vi "pdbm_TaskRoute_service.vi"(8 "error in (no error)":errorcluster, 10 "TaskDisplay":refnum<vi>, 11 "pdbm_testsys_event":T1) -> ()   [LabVIEW 2015]
doc: "handles message between pdbm_testsystem and tasks.\n-------------------------------------------------------------------\nAuthor: Dang Lam\nCreated: Feb, 10, 2012"
uses:
  pdbm_testsys_taskroute_inter/UsrDefine/pdbm_testsys_reqst_data.ctl
  test_system/UsrDefine/pdbm_testsystem_feedback_data.ctl
  test_system/public/getTaskInfo_byRef.vi
  pdbm_test_route/pdbm_task_route.lvlib
  test_system/pdbm_test_system.lvlib
  pdbm_testsys_taskroute_inter/pdbm_testsys_taskroute_inter.lvlib
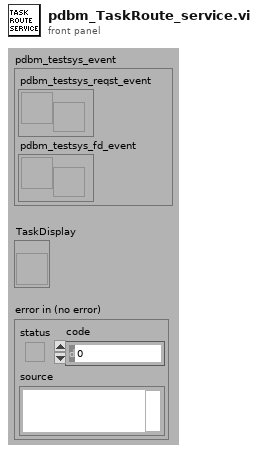
[diagram p1: front panel]
types:
  T1 = cluster{"pdbm_testsys_reqst_event":refnum<user-event>, "pdbm_testsys_fd_event":refnum<user-event>}
  T2 = cluster{"pdbm_testsys_reg_reqst_event":refnum<event-registration>, "pdbm_taskroute_reg_fd_event":refnum<event-registration>}
  T3 = cluster{"pdbm_testsys_fd_event":refnum<user-event>, "pdbm_testsys_reqst_event":refnum<user-event>, "pdbm_taskroute_fd_event":refnum<user-event>}
  T4 = cluster{"TaskName":string, "TaskRef":refnum<vi>}[]
  T5 = enum32{"Invalid", "Standard", "Closed", "Hidden", "Minimized", "Maximized"}
  T6 = typedef "pdbm_test_route.lvlib/TaskFeedbackCmd.ctl" = cluster{"TaskRef":refnum<vi>, "Command":string, "Variant":variant}
  T7 = typedef "pdbm_testsys_taskroute_inter.lvlib/pdbm_testsys_reqst_data.ctl" = cluster{"TaskName":string, "Request":string, "Data":variant}
  T8 = cluster{"pdbm_taskroute_fd_event":refnum<user-event>, "Data":variant}
  T9 = cluster{"TaskName":string, "Task Ref":refnum<vi>}
  T10 = cluster{"TaskName":string, "Task Ref":refnum<vi>}[]
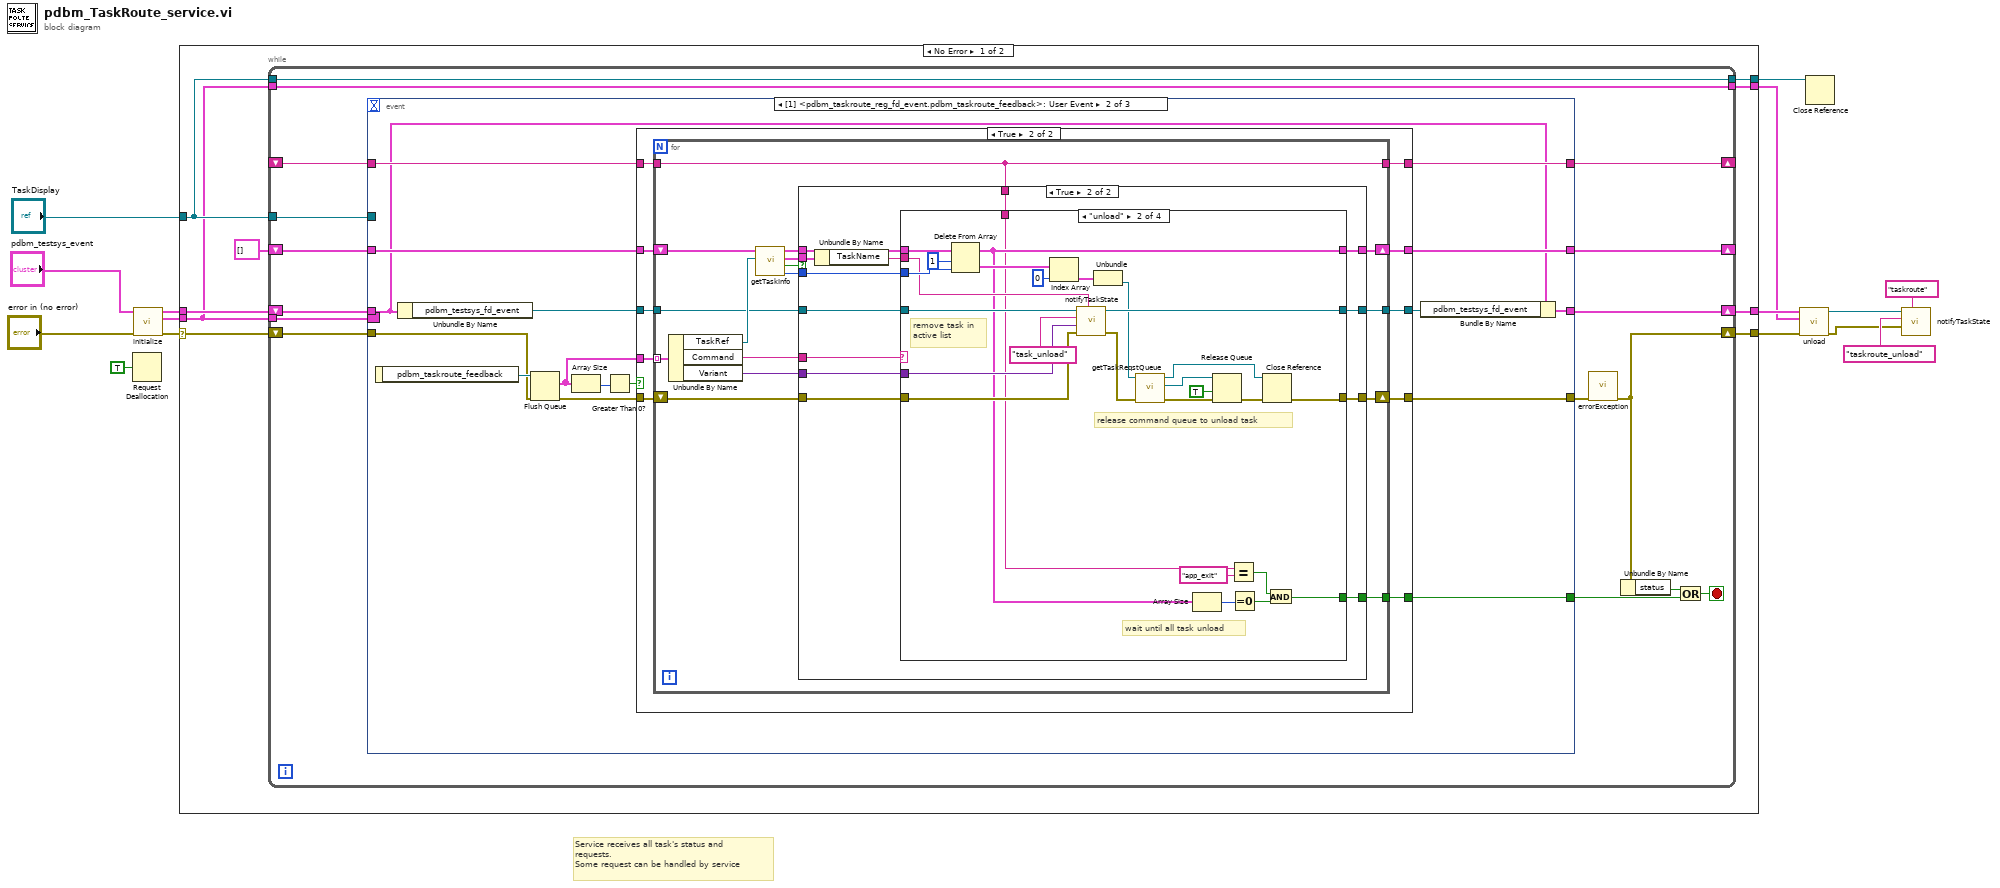
[diagram p0: block diagram]
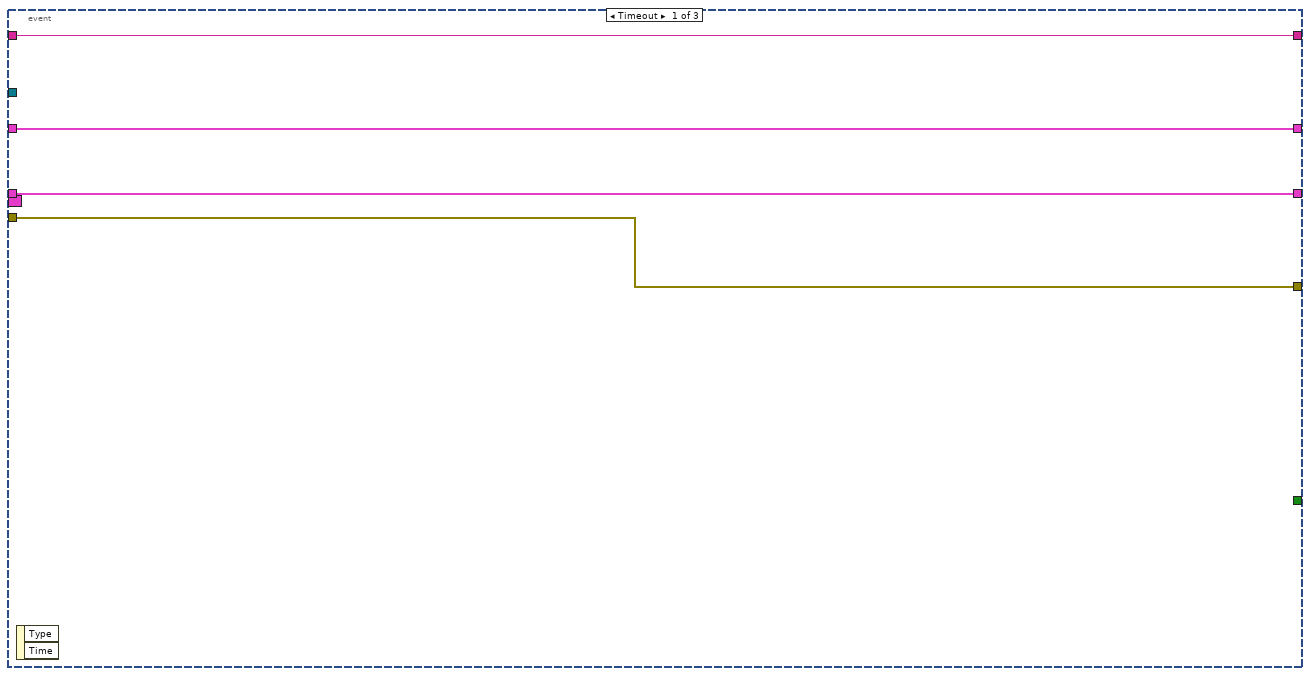
[diagram p2: hidden frame]
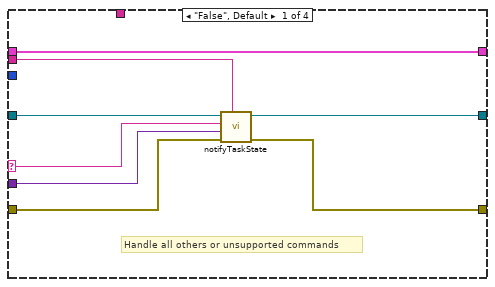
[diagram p5: hidden frame]
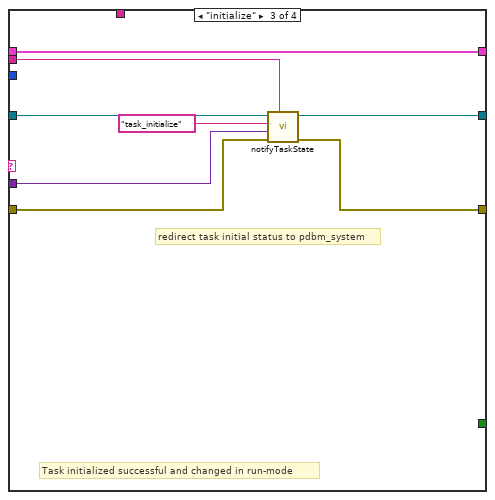
[diagram p6: hidden frame]
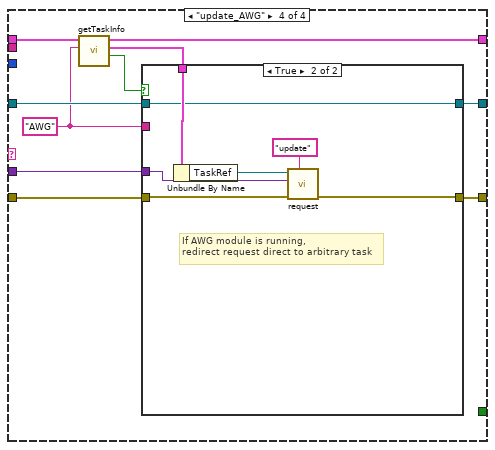
[diagram p7: hidden frame]
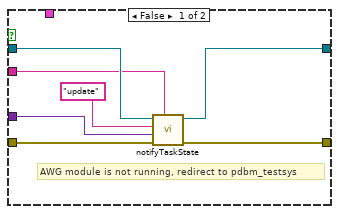
[diagram p8: hidden frame]
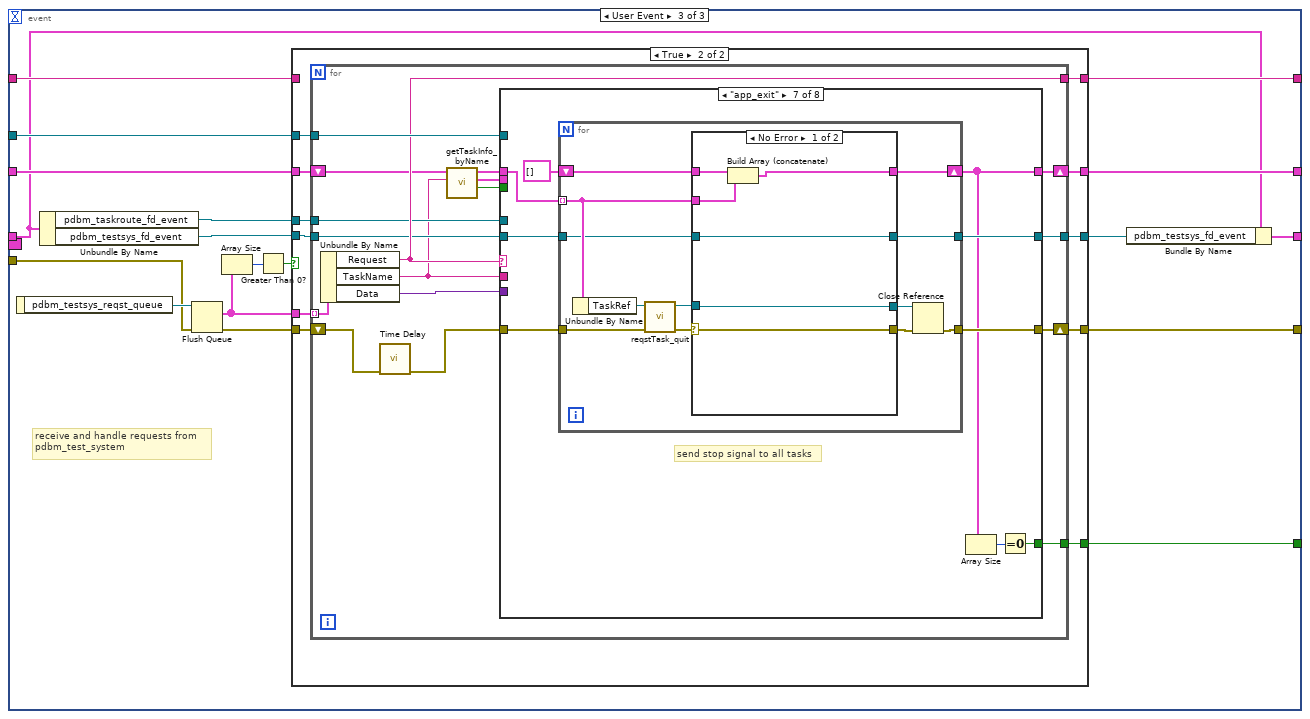
[diagram p9: hidden frame]
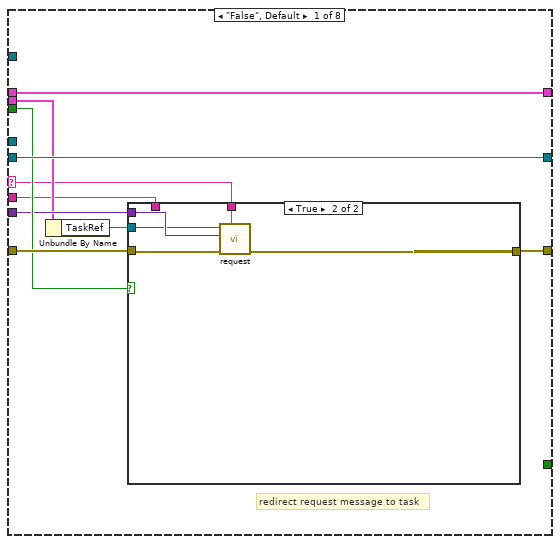
[diagram p11: hidden frame]
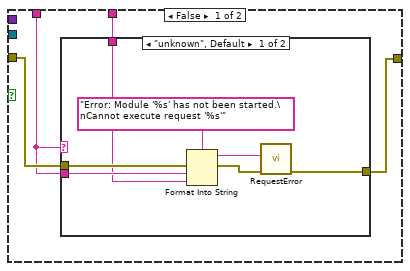
[diagram p12: hidden frame]
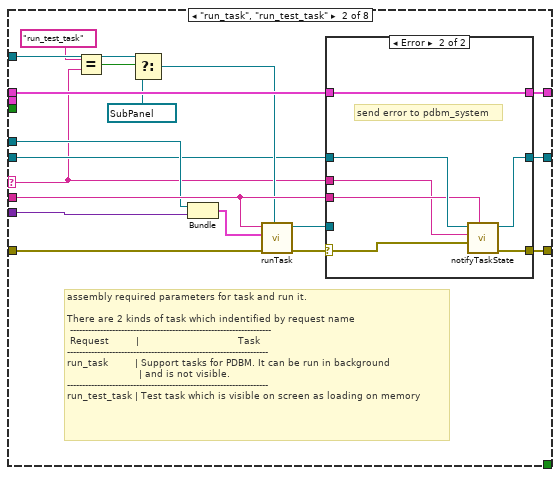
[diagram p14: hidden frame]
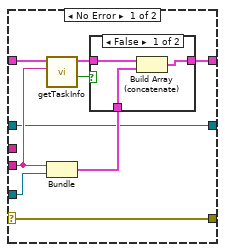
[diagram p15: hidden frame]
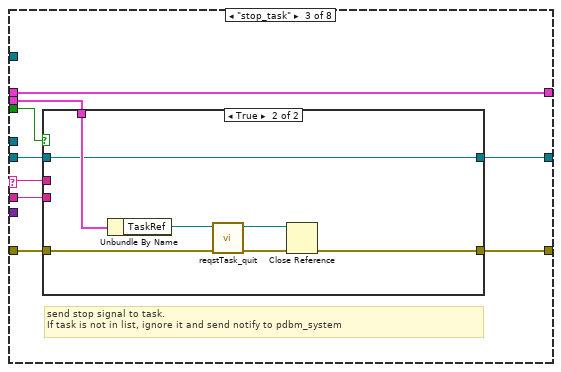
[diagram p17: hidden frame]
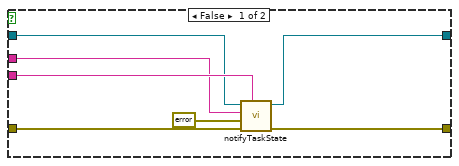
[diagram p18: hidden frame]
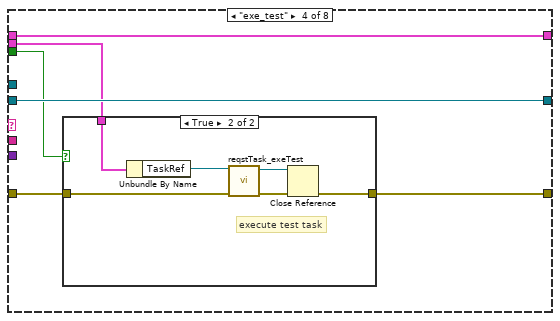
[diagram p19: hidden frame]
diagram:
  # "Service receives all task's status and\nrequests.\nSome request can be handled by service"
  n1 = Request Deallocation(TRUE ("flag")) -> ()
  n2 = call "initialize.vi"("error in (no error)"="error in (no error)", "pdbm_testsys_event"="pdbm_testsys_event") -> ("error IO"=w15:errorcluster, "pdbm_taskroute_reg_event"=w13:T2, "pdbm_taskroute_event"=w14:T3)  [unwired: 7 in]
  n3 = case shown="No Error" w15 {
    selector: w15 -> [w24 w381]
    tunnel: w14 -> [w21 w380]
    tunnel: w13 -> [w16 w379]
    tunnel: "TaskDisplay" -> [w20 w382]
    tunnel: [w19 w382] -> w2
    tunnel: [w22 w381] -> w7
    tunnel: [w18 w380] -> w6
    tunnel: [w17 w379] -> w5
    frame No Error {
      n4 = while {
        shift-right: [w27] -> w22
        shift-left: w24 -> [w40]
        tunnel: w16 -> [w39]
        shift-right: [w37] -> _
        shift-left: T4 [] -> [w38]
        tunnel: w20 -> [w36]
        shift-right: [w35] -> _
        shift-left: _ -> [w34]
        tunnel: w20 -> [w33]
        tunnel: [w33] -> w19
        shift-right: [w28] -> w18
        shift-left: w21 -> [w26]
        tunnel: [w25] -> w17
        tunnel: w16 -> [w25]
        stop <- w30 stop-if-true
        n5 = event shown="[1] <pdbm_taskroute_reg_fd_event.pdbm_taskroute_feedback>: User Event" {
          selector: w39 -> [_ _ _]
          dyn-events: _ -> [_ _ _]
          timeout: _ -> [_ _ _]
          tunnel: w40 -> [w43 w59 w190]
          tunnel: [w43 w58 w188] -> w32
          tunnel: w38 -> [w44 w57 w187]
          tunnel: [w44 w56 w186] -> w37
          tunnel: w36 -> [_ _ w185]
          tunnel: [w42 w54 w184] -> w35
          tunnel: w34 -> [w42 w55 w180]
          tunnel: [_ w53 w179] -> w31
          tunnel: w26 -> [w41 w47 w177]
          tunnel: [w41 w46 w175] -> w28
          event Timeout {
            n6 = event-data() -> ()  [unwired: 1 in, 2 out]
          }
          event User Event {
            n7 = event-data() -> ("pdbm_taskroute_feedback"=w60:refnum<queue>)  [unwired: 1 in]
            n8 = Unbundle By Name(w47) -> ("pdbm_testsys_fd_event"=w52:refnum<user-event>)
            n9 = Flush Queue(queue=w60, error in (no error)=w59) -> (remaining elements=w51:T6[], error out=w48:errorcluster)  [unwired: 1 out]
            n10 = Array Size(array=w51) -> (size(s)=w49:i32)
            n11 = Greater Than 0?(x=w49) -> (x > 0?=w50:bool)
            n12 = case shown="True" w50 {
              tunnel: w51 -> [_ w74]
              tunnel: [w61 w73] -> w58
              tunnel: w57 -> [w63 w72]
              tunnel: [w63 w71] -> w56
              tunnel: w55 -> [w64 w70]
              tunnel: [w64 w69] -> w54
              tunnel: [_ w68] -> w53
              tunnel: w52 -> [w62 w67]
              tunnel: [w62 w66] -> w45
              tunnel: w48 -> [w61 w65]
              frame False {
              }
              frame True {
                n13 = for {
                  tunnel: w74 -> [w89] mode=indexing
                  shift-right: [w80] -> w73
                  shift-left: w65 -> [w75]
                  shift-right: [w81] -> w71
                  shift-left: w72 -> [w90]
                  tunnel: w70 -> [w79]
                  tunnel: [w79] -> w69
                  tunnel: [w78] -> w68
                  tunnel: w67 -> [w77]
                  tunnel: [w76] -> w66
                  n14 = Unbundle By Name(w89) -> ("TaskRef"=w88:refnum<vi>, "Command"=w83:string, "Variant"=w82:variant)
                  n15 = call-poly "getTaskInfo.vi"("TaskRef in"=w88, "ActiveTask in"=w90) -> ("index"=w84:i32, "found?"=w87:bool, "TaskInfo"=w85:cluster{"TaskName":string, "TaskRef":refnum<vi>}, "ActiveTask out"=w86:T4)  [unwired: 6 in]
                  n16 = case shown="True" w87 {
                    tunnel: w86 -> [w93 w106]
                    tunnel: w85 -> [_ w95]
                    tunnel: w84 -> [_ w104]
                    tunnel: w83 -> [_ w105]
                    tunnel: w82 -> [_ w102]
                    tunnel: [w93 w103] -> w81
                    tunnel: w75 -> [w92 w101]
                    tunnel: [w92 w100] -> w80
                    tunnel: w79 -> [_ w99]
                    tunnel: [_ w98] -> w78
                    tunnel: w77 -> [w91 w97]
                    tunnel: [w91 w96] -> w76
                    frame False {
                    }
                    frame True {
                      n17 = Unbundle By Name(w95) -> ("TaskName"=w94:string)
                      n18 = case shown="\"unload\"" w105 {
                        selector: w105 -> [w110 _ _ _]
                        tunnel: w106 -> [w114 w141 w149 w159]
                        tunnel: w104 -> [_ w140 _ _]
                        tunnel: [w114 w116 w149 w158] -> w103
                        tunnel: w102 -> [w112 w133 w148 w152]
                        tunnel: [w109 w119 w146 w153] -> w100
                        tunnel: w101 -> [w111 w134 w147 w154]
                        tunnel: w99 -> [_ w115 _ _]
                        tunnel: [_ w136 _ _] -> w98
                        tunnel: w97 -> [w113 w135 w145 w156]
                        tunnel: w94 -> [w107 w130 w142 _]
                        tunnel: [w108 w131 w143 w151] -> w96
                        frame "False", Default {
                          # "Handle all others or unsupported commands"
                          n19 = call "notifyTaskState.vi"("TaskName"=w107, "error in (no error)"=w111, "Data"=w112, "Request"=w110, "pdbm_testsystem_feeback_event"=w113) -> ("error out"=w109:errorcluster, "pdbm_testsystem_feeback_event out"=w108:refnum<user-event>)  [unwired: 5 in]
                        }
                        frame "unload" {
                          # "release command queue to unload task"
                          # "remove task in\nactive list"
                          # "wait until all task unload"
                          n20 = Delete From Array(array=w141, length=1, index=w140) -> (deleted portion=w124:T4, array with subset deleted=w116:T4)
                          n21 = Index Array(array=w124, index=0) -> (element=w125:cluster{"TaskName":string, "TaskRef":refnum<vi>})
                          n22 = call "notifyTaskState.vi"("TaskName"=w130, "error in (no error)"=w134, "Data"=w133, "Request"="task_unload", "pdbm_testsystem_feeback_event"=w135) -> ("error out"=w126:errorcluster, "pdbm_testsystem_feeback_event out"=w131:refnum<user-event>)  [unwired: 5 in]
                          n23 = Unbundle(w125) -> ("TaskRef"=w123:refnum<vi>)  [unwired: 1 out]
                          n24 = call "getTaskReqstQueue.vi"("error in (no error)"=w126, "TaskRef"=w123) -> ("error IO"=w122:errorcluster, "TaskReqst_queue"=w121:refnum<queue>, "TaskRef out"=w118:refnum<vi>)  [unwired: 7 in]
                          n25 = Array Size(array=w116) -> (size(s)=w137:i32)
                          n26 = Release Queue(queue=w121, force destroy? (F)=TRUE, error in (no error)=w122) -> (error out=w120:errorcluster)  [unwired: 2 out]
                          n27 = Equal?(x=w115, y="app_exit") -> (x = y?=w127:bool)
                          n28 = Equal To 0?(x=w137) -> (x = 0?=w128:bool)
                          n29 = Close Reference(reference=w118, error in (no error)=w120) -> (error out=w119:errorcluster)
                          n30 = And(x=w127, y=w128) -> (x .and. y?=w136:bool)
                        }
                        frame "initialize" {
                          # "redirect task initial status to pdbm_system"
                          # "Task initialized successful and changed in run-mode"
                          n31 = call "notifyTaskState.vi"("TaskName"=w142, "error in (no error)"=w147, "Data"=w148, "Request"="task_initialize", "pdbm_testsystem_feeback_event"=w145) -> ("error out"=w146:errorcluster, "pdbm_testsystem_feeback_event out"=w143:refnum<user-event>)  [unwired: 5 in]
                        }
                        frame "update_AWG" {
                          w150 = "AWG" ("TaskName")
                          n32 = call-poly "getTaskInfo.vi"("TaskName"=w150, "ActiveTask in"=w159) -> ("found?"=w157:bool, "TaskInfo"=w155:cluster{"TaskName":string, "TaskRef":refnum<vi>}, "ActiveTask out"=w158:T4)  [unwired: 6 in, 1 out]
                          n33 = case shown="True" w157 {
                            tunnel: w156 -> [w166 w167]
                            tunnel: w155 -> [_ w170]
                            tunnel: w154 -> [w164 w173]
                            tunnel: [w163 w172] -> w153
                            tunnel: w152 -> [w160 w168]
                            tunnel: [w165 w167] -> w151
                            tunnel: w150 -> [w162 _]
                            frame False {
                              # "AWG module is not running, redirect to pdbm_testsys"
                              n34 = call "notifyTaskState.vi"("TaskName"=w162, "error in (no error)"=w164, "Data"=w160, "Request"="update", "pdbm_testsystem_feeback_event"=w166) -> ("error out"=w163:errorcluster, "pdbm_testsystem_feeback_event out"=w165:refnum<user-event>)  [unwired: 5 in]
                            }
                            frame True {
                              # "If AWG module is running,\nredirect request direct to arbitrary task"
                              n35 = Unbundle By Name(w170) -> ("TaskRef"=w169:refnum<vi>)
                              n36 = call "request.vi"("request"="update", "error in (no error)"=w173, "Parameter"=w168, "TaskRef in"=w169) -> ("error IO"=w172:errorcluster)  [unwired: 6 in, 1 out]
                            }
                          }
                        }
                      }
                    }
                  }
                }
              }
            }
            n37 = Bundle By Name(cluster=w47, "pdbm_testsys_fd_event"=w45) -> (w46:T3)
          }
          event User Event {
            # "receive and handle requests from\npdbm_test_system"
            n38 = event-data() -> ("pdbm_testsys_reqst_queue"=w191:refnum<queue>)  [unwired: 1 in]
            n39 = Unbundle By Name(w177) -> ("pdbm_taskroute_fd_event"=w174:refnum<user-event>, "pdbm_testsys_fd_event"=w178:refnum<user-event>)
            n40 = Flush Queue(queue=w191, error in (no error)=w190) -> (remaining elements=w183:T7[], error out=w189:errorcluster)  [unwired: 1 out]
            n41 = Array Size(array=w183) -> (size(s)=w182:i32)
            n42 = Greater Than 0?(x=w182) -> (x > 0?=w181:bool)
            n43 = case shown="True" w181 {
              tunnel: w189 -> [w193 w206]
              tunnel: [w193 w205] -> w188
              tunnel: w178 -> [w192 w204]
              tunnel: w187 -> [w194 w203]
              tunnel: [w194 w202] -> w186
              tunnel: w185 -> [_ w201]
              tunnel: [w195 w200] -> w184
              tunnel: w183 -> [_ w199]
              tunnel: w180 -> [w195 _]
              tunnel: [_ w198] -> w179
              tunnel: [w192 w197] -> w176
              tunnel: w174 -> [_ w196]
              frame False {
              }
              frame True {
                n44 = for {
                  tunnel: w199 -> [w223] mode=indexing
                  shift-right: [w221] -> w205
                  shift-left: w206 -> [w208]
                  tunnel: w204 -> [w216]
                  shift-right: [w220] -> w202
                  shift-left: w203 -> [w213]
                  tunnel: w201 -> [w219]
                  tunnel: [w218] -> w200
                  tunnel: [w217] -> w198
                  tunnel: [w215] -> w197
                  tunnel: w196 -> [w214]
                  n45 = Unbundle By Name(w223) -> ("Request"=w218:string, "TaskName"=w211:string, "Data"=w222:variant)
                  n46 = call "Time Delay"("error in (no error)"=w208) -> ("error out"=w207:errorcluster)  [unwired: 10 in]
                  n47 = call "getTaskInfo_byName.vi"("TaskName"=w211, "ActiveTask in"=w213) -> ("found?"=w209:bool, "TaskInfo"=w210:cluster{"TaskName":string, "TaskRef":refnum<vi>}, "ActiveTask out"=w212:T4)  [unwired: 6 in, 1 out]
                  n48 = case shown="\"app_exit\"" w218 {
                    selector: w218 -> [w225 w251 w294 _ _ _ _ _]
                    tunnel: w216 -> [w233 w253 w293 w315 w325 w328 w334 w367]
                    tunnel: w207 -> [w231 w268 w297 w317 w327 w330 w339 w371]
                    tunnel: w211 -> [w224 w263 w295 _ _ _ _ _]
                    tunnel: w222 -> [w229 w267 _ _ _ _ _ _]
                    tunnel: [w228 w265 w296 w316 w327 w330 w338 w370] -> w221
                    tunnel: w212 -> [w232 w264 w291 w314 w326 w329 w335 w369]
                    tunnel: [w232 w261 w291 w314 w326 w329 w332 w368] -> w220
                    tunnel: w219 -> [_ w260 _ _ _ _ _ _]
                    tunnel: [_ _ _ _ _ _ w336 _] -> w217
                    tunnel: [w233 w252 w292 w315 w325 w328 w333 w367] -> w215
                    tunnel: w214 -> [_ w254 _ _ _ _ _ _]
                    tunnel: w210 -> [w227 _ w290 w313 _ _ _ _]
                    tunnel: w209 -> [w230 _ w289 w312 _ _ _ _]
                    frame "False", Default {
                      # "redirect request message to task"
                      n49 = Unbundle By Name(w227) -> ("TaskRef"=w226:refnum<vi>)
                      n50 = case shown="True" w230 {
                        tunnel: w231 -> [w237 w250]
                        tunnel: w229 -> [_ w248]
                        tunnel: [w235 w249] -> w228
                        tunnel: w226 -> [_ w247]
                        tunnel: w225 -> [w236 w246]
                        tunnel: w224 -> [w234 _]
                        frame False {
                          n51 = case shown="\"unknown\", Default" w234 {
                            tunnel: w234 -> [w243 _]
                            tunnel: w237 -> [w242 w245]
                            tunnel: w236 -> [w241 _]
                            tunnel: [w238 w245] -> w235
                            frame "unknown", Default {
                              n52 = Format Into String(format string="Error: Module '%s' has not been started.\nCannot execute request '%s'", error in=w242, w243, w241) -> (resulting string=w240:string, error out=w239:errorcluster)  [unwired: 1 in]
                              n53 = call "RequestError"("error in (no error)"=w239, "Message"=w240) -> ("error out"=w238:errorcluster)  [unwired: 8 in, 1 out]
                            }
                            frame "Config_Test_Sequence", "HrdwareConfig" {
                            }
                          }
                        }
                        frame True {
                          n54 = call "request.vi"("request"=w246, "error in (no error)"=w250, "Parameter"=w248, "TaskRef in"=w247) -> ("error IO"=w249:errorcluster)  [unwired: 6 in, 1 out]
                        }
                      }
                    }
                    frame "run_task", "run_test_task" {
                      # "assembly required parameters for task and run it.\n\nThere are 2 kinds of task which indentified by request name\n -------------------------------------------------------------------\n Request         |                                 Task\n-------------------------------------------------------------------\nrun_task         | Support tasks for PDBM. It can be run in background\n                        | and is not visible.\n-------------------------------------------------------------------\nrun_test_task | Test task which is visible on screen as loading on memory"
                      n55 = Equal?(x="run_test_task", y=w251) -> (x = y?=w259:bool)
                      n56 = Select(t=w260, s=w259, f=refnum<vi> refnum) -> (s? t:f=w257:refnum<vi>)
                      n57 = Bundle("pdbm_taskroute_fd_event"=w254, "Data"=w267) -> (w256:T8)  [unwired: 1 in]
                      n58 = call "runTask.vi"("SubPanel Ref"=w257, "error in (no error)"=w268, "Parameter"=w256, "Taskname"=w263) -> ("error out"=w266:errorcluster, "Task Ref"=w262:refnum<vi>)  [unwired: 6 in]
                      n59 = case shown="Error" w266 {
                        selector: w266 -> [w277 w287]
                        tunnel: [w277 w286] -> w265
                        tunnel: w264 -> [w273 w288]
                        tunnel: w263 -> [w271 w283]
                        tunnel: w262 -> [w276 _]
                        tunnel: [w274 w288] -> w261
                        tunnel: w253 -> [w269 w285]
                        tunnel: [w269 w284] -> w252
                        tunnel: w251 -> [_ w282]
                        frame No Error {
                          n60 = call-poly "getTaskInfo.vi"("TaskName"=w271, "ActiveTask in"=w273) -> ("found?"=w270:bool, "ActiveTask out"=w272:T4)  [unwired: 6 in, 2 out]
                          n61 = Bundle("TaskName"=w271, "Task Ref"=w276) -> (w275:T9)  [unwired: 1 in]
                          n62 = case shown="False" w270 {
                            tunnel: w275 -> [w280 _]
                            tunnel: [w279 w281] -> w274
                            tunnel: w272 -> [w278 w281]
                            frame False {
                              n63 = Build Array (concatenate)(w278, w280) -> (w279:T10)
                            }
                            frame True {
                            }
                          }
                        }
                        frame Error {
                          # "send error to pdbm_system"
                          n64 = call "notifyTaskState.vi"("TaskName"=w283, "Data"=w287, "Request"=w282, "pdbm_testsystem_feeback_event"=w285) -> ("error out"=w286:errorcluster, "pdbm_testsystem_feeback_event out"=w284:refnum<user-event>)  [unwired: 6 in]
                        }
                      }
                    }
                    frame "stop_task" {
                      # "send stop signal to task.\nIf task is not in list, ignore it and send notify to pdbm_system"
                      n65 = case shown="True" w289 {
                        tunnel: w297 -> [w304 w311]
                        tunnel: [w303 w308] -> w296
                        tunnel: w290 -> [_ w307]
                        tunnel: w295 -> [w302 _]
                        tunnel: w294 -> [w301 _]
                        tunnel: w293 -> [w299 w305]
                        tunnel: [w298 w305] -> w292
                        frame False {
                          n66 = call "notifyTaskState.vi"("TaskName"=w302, "error in (no error)"=w304, "Data"=errorcluster {"status"=TRUE, "code"=0, "source"="Task does not exist in active list"} ("error out"), "Request"=w301, "pdbm_testsystem_feeback_event"=w299) -> ("error out"=w303:errorcluster, "pdbm_testsystem_feeback_event out"=w298:refnum<user-event>)  [unwired: 5 in]
                        }
                        frame True {
                          n67 = Unbundle By Name(w307) -> ("TaskRef"=w306:refnum<vi>)
                          n68 = call "reqstTask_quit.vi"("error in (no error)"=w311, "TaskRef in"=w306) -> ("error IO"=w310:errorcluster, "TaskRef out"=w309:refnum<vi>)  [unwired: 8 in]
                          n69 = Close Reference(reference=w309, error in (no error)=w310) -> (error out=w308:errorcluster)
                        }
                      }
                    }
                    frame "exe_test" {
                      n70 = case shown="True" w312 {
                        tunnel: w313 -> [_ w320]
                        tunnel: w317 -> [w318 w324]
                        tunnel: [w318 w321] -> w316
                        frame False {
                        }
                        frame True {
                          # "execute test task"
                          n71 = Unbundle By Name(w320) -> ("TaskRef"=w319:refnum<vi>)
                          n72 = call "reqstTask_exeTest.vi"("error in (no error)"=w324, "TaskRef in"=w319) -> ("error IO"=w323:errorcluster, "TaskRef out"=w322:refnum<vi>)  [unwired: 8 in]
                          n73 = Close Reference(reference=w322, error in (no error)=w323) -> (error out=w321:errorcluster)
                        }
                      }
                    }
                    frame "halt_test" {
                    }
                    frame "stop_test" {
                      # "run new task and assembly it on panel"
                    }
                    frame "app_exit" {
                      # "send stop signal to all tasks"
                      n74 = for {
                        tunnel: w339 -> [w351]
                        tunnel: w335 -> [w343] mode=indexing
                        tunnel: [w345] -> w338
                        shift-right: [w342] -> w332
                        shift-left: T4 [] ("appended array") -> [w344]
                        tunnel: w334 -> [w341]
                        tunnel: [w340] -> w333
                        n75 = Unbundle By Name(w343) -> ("TaskRef"=w350:refnum<vi>)
                        n76 = call "reqstTask_quit.vi"("error in (no error)"=w351, "TaskRef in"=w350) -> ("error IO"=w349:errorcluster, "TaskRef out"=w348:refnum<vi>)  [unwired: 8 in]
                        n77 = case shown="No Error" w349 {
                          selector: w349 -> [w357 _]
                          tunnel: w348 -> [w356 w364]
                          tunnel: [w356 w366] -> w346
                          tunnel: [w357 w365] -> w347
                          tunnel: w344 -> [w355 w359]
                          tunnel: w343 -> [w354 _]
                          tunnel: [w353 w359] -> w342
                          tunnel: w341 -> [w352 w358]
                          tunnel: [w352 w358] -> w340
                          frame No Error {
                            n78 = Build Array (concatenate)(w355, w354) -> (w353:T4)
                          }
                          frame Error {
                            n79 = invoke class="VI" method="FP.Open"(reference=w364, "Activate"=TRUE ("Activate?"), "State"=T5."Standard") -> (reference out=w363:refnum<vi>, error out=w362:errorcluster)  [unwired: 2 in, 3 out]
                            n80 = invoke class="VI" method="FP.Close"(reference=w363, error in=w362) -> (reference out=w366:refnum<vi>, error out=w365:errorcluster)  [unwired: 1 in, 1 out]
                          }
                        }
                        n81 = Close Reference(reference=w346, error in (no error)=w347) -> (error out=w345:errorcluster)
                      }
                      n82 = Array Size(array=w332) -> (size(s)=w337:i32)
                      n83 = Equal To 0?(x=w337) -> (x = 0?=w336:bool)
                    }
                    frame "ReInit" {
                      # "send stop signal to all tasks"
                      n84 = for {
                        tunnel: w371 -> [w375]
                        tunnel: w369 -> [w377] mode=indexing
                        tunnel: [w378] -> w370
                        tunnel: [w377] -> w368 mode=indexing
                        n85 = Unbundle By Name(w377) -> ("TaskRef"=w376:refnum<vi>)
                        n86 = call "request.vi"("request"="ReInit", "error in (no error)"=w375, "TaskRef in"=w376) -> ("error IO"=w374:errorcluster, "TaskRef out"=w373:refnum<vi>)  [unwired: 7 in]
                        n87 = Close Reference(reference=w373, error in (no error)=w374) -> (error out=w378:errorcluster)
                      }
                    }
                  }
                }
              }
            }
            n88 = Bundle By Name(cluster=w177, "pdbm_testsys_fd_event"=w176) -> (w175:T3)
          }
        }
        n89 = call "errorException.vi"("error in (no error)"=w32) -> ("error IO"=w27:errorcluster)  [unwired: 10 in]
        n90 = Unbundle By Name(w27) -> ("status"=w29:bool)
        n91 = Or(x=w29, y=w31) -> (x .or. y?=w30:bool)
      }
    }
    frame Error {
    }
  }
  n92 = call "unload.vi"("error in (no error)"=w7, "pdbm_taskroute_reg_event"=w5, "pdbm_taskroute_event"=w6) -> ("error out"=w4:errorcluster, "pdbm_testsys_fd_event"=w3:refnum<user-event>)  [unwired: 7 in]
  n93 = Close Reference(reference=w2) -> ()  [unwired: 1 in, 1 out]
  n94 = call "notifyTaskState.vi"("TaskName"="taskroute", "Data"=w4, "Request"="taskroute_unload", "pdbm_testsystem_feeback_event"=w3) -> ()  [unwired: 6 in, 2 out]
